vi "Popup window-Cursor value entry.vi"(7 "Waveform Ref in":T3, 10 "Xinformation In":T1, 11 "Timeline Ref in":T5) -> (0 "error out":errorcluster, 1 "Cancelled":bool, 2 "Xinformation Out":T1={"Cursor Span"=0.0, "Icon"=0, "Mouse Down"=FALSE, "Owning VI"=refnum, "Mouse area"=enum."Move", "Dragging"=FALSE, "Drag Offset"=0.0, "Original Cursor Pos"={"Left"=0.0, "Right"=0.0, "Span"=0.0}, "Cursor Redraw"=TRUE}, 3 "Timeline Ref out":T5)   [LabVIEW 2013, in "XGrapher.xctl"]
uses:
  XGrapher.xctl
  Typedefs/Xctrl-Timeline graph ref.ctl
  Typedefs/Xinformation.ctl
  Typedefs/Xcrtl-Click Operation.ctl
  Typedefs/Xctrl-Waveform graph ref.ctl
panel:
  out "Timeline Graph":T4(graph)
  in  "Right Cursor (sec)":dbl min=0.005864328141225338 max=0.085028
  in  "Left Cursor (sec)":dbl min=0.0 max=0.06454358047767395
  in  "Cancel":bool
  in  "OK":bool
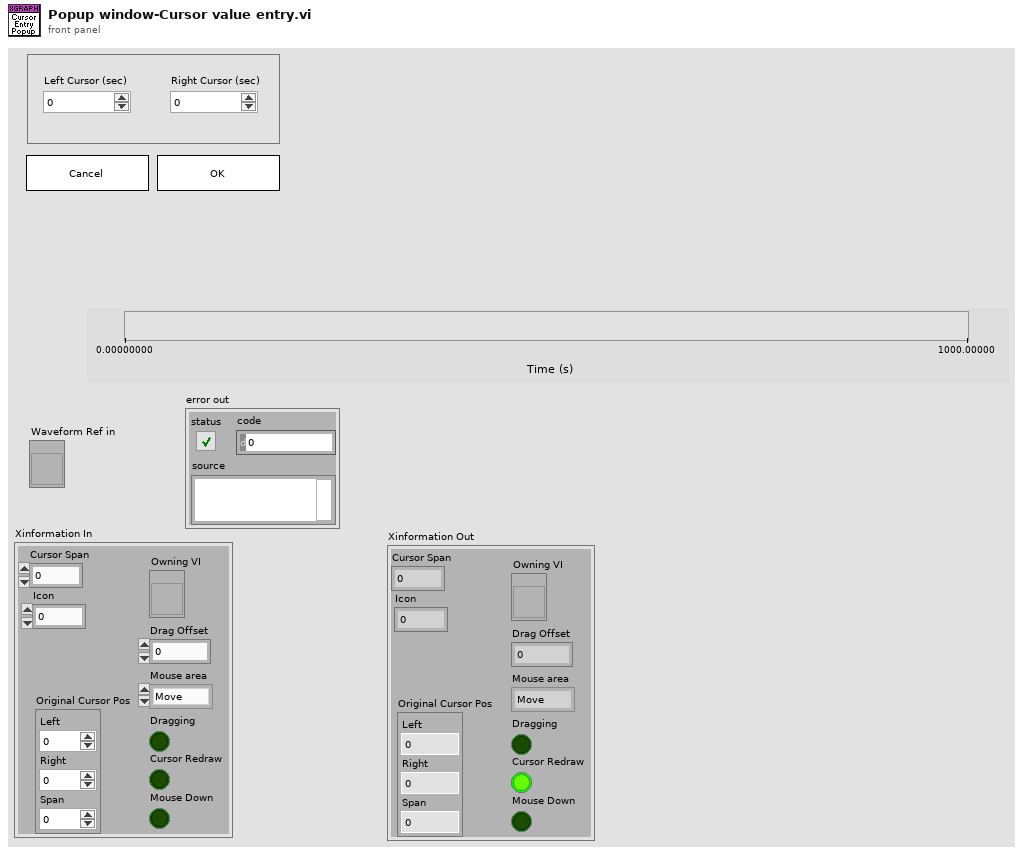
[diagram p1: front panel]
types:
  T1 = typedef "XGrapher.xctl/Xinformation.ctl" = cluster{"Cursor Span":dbl, "Icon":u16, "Mouse Down":bool, "Owning VI":refnum<vi>, "Mouse area":T2, "Dragging":bool, "Drag Offset":dbl, "Original Cursor Pos":cluster{"Left":dbl, "Right":dbl, "Span":dbl}, "Cursor Redraw":bool}
  T2 = typedef "XGrapher.xctl/Xcrtl-Click Operation.ctl" = enum16{"Move", "left cursor", "right cursor", "none"}
  T3 = typedef "XGrapher.xctl/Xctrl-Waveform graph ref.ctl" = refnum<vi>
  T4 = cluster{"X-Axis values":dbl[], "Y-Axis values":dbl[]}[]
  T5 = typedef "XGrapher.xctl/Xctrl-Timeline graph ref.ctl" = refnum<vi>
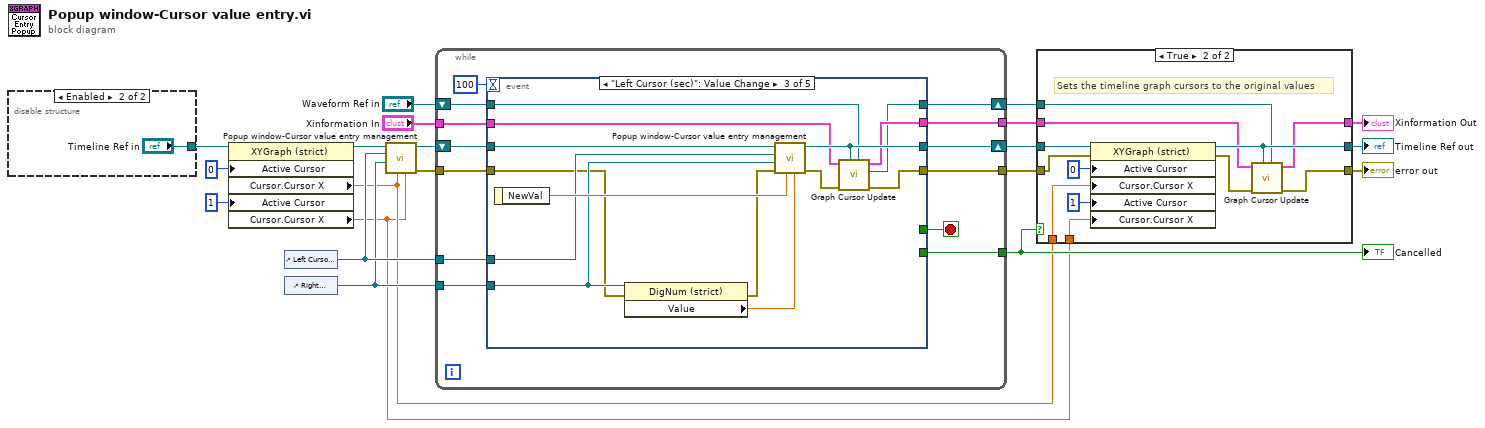
[diagram p0: block diagram]
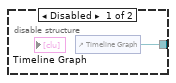
[diagram p3: hidden frame]
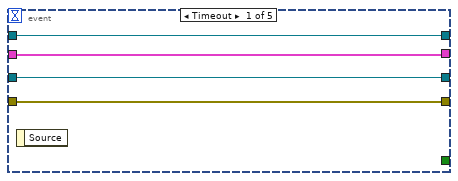
[diagram p4: hidden frame]
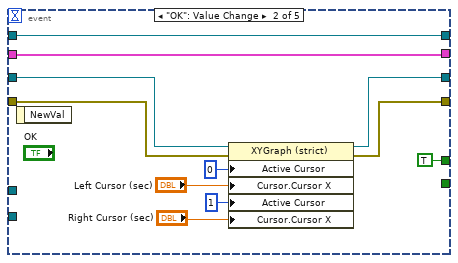
[diagram p5: hidden frame]
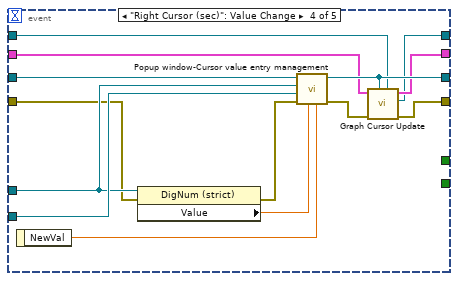
[diagram p6: hidden frame]
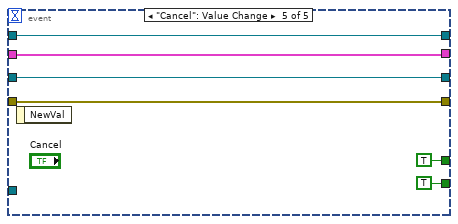
[diagram p7: hidden frame]
diagram:
  n1 = disable-structure shown="Enabled" {
    disable-tunnel: [w21 "Timeline Ref in"] -> w13
    frame Disabled {
      n2 = control-ref of="Timeline Graph"() -> (w21:refnum<vi>)
    }
    frame Enabled {
    }
  }
  n3 = property on="Property Node" class="XYGraph (strict)"(reference=w13, "Active Cursor"=u32 0, "Active Cursor"=u32 1) -> (reference out=w14:T5, "Cursor.Cursor X"=w8:dbl, "Cursor.Cursor X"=w7:dbl)  [unwired: 1 in, 1 out]
  n4 = control-ref of="Left Cursor (sec)"() -> (w18:refnum<vi>)
  n5 = control-ref of="Right Cursor (sec)"() -> (w17:refnum<vi>)
  n6 = call "Popup window-Cursor value entry management.vi"("Rightcursor position"=w7, "Left cursor position"=w8, "Right control ref"=w17, "Left control ref"=w18, "Timeline Ref in"=w14) -> ("error out"=w19:errorcluster, "XYGraph out"=w20:T5)  [unwired: 5 in]
  n7 = while {
    tunnel: [w33] -> w12
    tunnel: w19 -> [w31]
    tunnel: [w30] -> w11
    tunnel: w18 -> [w29]
    tunnel: w17 -> [w28]
    tunnel: "Xinformation In" -> [w26]
    tunnel: [w25] -> w2
    shift-right: [w24] -> w4
    shift-left: w20 -> [w32]
    shift-right: [w23] -> w3
    shift-left: "Waveform Ref in" -> [w27]
    stop <- w34 stop-if-true
    n8 = event shown="[2] \"Left Cursor (sec)\": Value Change" {
      selector: _ -> [_ _ _ _ _]
      dyn-events: _ -> [_ _ _ _ _]
      timeout: 100 -> [_ _ _ _ _]
      tunnel: [_ TRUE ("Cancel") _ _ TRUE ("Cancel")] -> w34
      tunnel: [_ _ _ _ TRUE ("Cancel")] -> w33
      tunnel: w32 -> [w39 w46 w64 w78 w84]
      tunnel: [w39 w45 w57 w69 w84] -> w24
      tunnel: w31 -> [w38 w43 w59 w73 w81]
      tunnel: [w38 w42 w52 w70 w81] -> w30
      tunnel: w29 -> [_ _ w62 w74 _]
      tunnel: w28 -> [_ _ w61 w77 _]
      tunnel: w27 -> [w36 w40 w56 w68 w79]
      tunnel: w26 -> [w37 w41 w55 w67 w80]
      tunnel: [w37 w41 w54 w66 w80] -> w25
      tunnel: [w36 w40 w51 w65 w79] -> w23
      event Timeout {
        n9 = event-data() -> ()  [unwired: 1 in, 1 out]
      }
      event "OK": Value Change {
        n10 = event-data() -> ()  [unwired: 1 in, 1 out]
        n11 = property class="XYGraph (strict)"(reference=w46, error in=w43, "Active Cursor"=u32 0, "Cursor.Cursor X"="Left Cursor (sec)", "Active Cursor"=u32 1, "Cursor.Cursor X"="Right Cursor (sec)") -> (reference out=w45:T5, error out=w42:errorcluster)
      }
      event "Left Cursor (sec)": Value Change {
        n12 = event-data() -> ("NewVal"=w63:dbl)  [unwired: 1 in]
        n13 = property on="Property Node" class="DigNum (strict)"(reference=w61, error in=w59) -> (error out=w58:errorcluster, "Value"=w60:dbl)  [unwired: 1 out]
        n14 = call "Popup window-Cursor value entry management.vi"("Rightcursor position"=w60, "Left cursor position"=w63, "error in"=w58, "Right control ref"=w61, "Left control ref"=w62, "Timeline Ref in"=w64) -> ("error out"=w53:errorcluster, "XYGraph out"=w57:T5)  [unwired: 4 in]
        n15 = call "Graph Cursor Update.vi"("Waveform Ref in"=w56, "Timeline Ref in"=w57, "error in (no error)"=w53, "Xinformation In"=w55) -> ("error out"=w52:errorcluster, "Waveform Ref out"=w51:T3, "Xinformation Out"=w54:T1)  [unwired: 5 in]
      }
      event "Right Cursor (sec)": Value Change {
        n16 = event-data() -> ("NewVal"=w76:dbl)  [unwired: 1 in]
        n17 = property on="Property Node" class="DigNum (strict)"(reference=w74, error in=w73) -> (error out=w72:errorcluster, "Value"=w75:dbl)  [unwired: 1 out]
        n18 = call "Popup window-Cursor value entry management.vi"("Rightcursor position"=w76, "Left cursor position"=w75, "error in"=w72, "Right control ref"=w77, "Left control ref"=w74, "Timeline Ref in"=w78) -> ("error out"=w71:errorcluster, "XYGraph out"=w69:T5)  [unwired: 4 in]
        n19 = call "Graph Cursor Update.vi"("Waveform Ref in"=w68, "Timeline Ref in"=w69, "error in (no error)"=w71, "Xinformation In"=w67) -> ("error out"=w70:errorcluster, "Waveform Ref out"=w65:T3, "Xinformation Out"=w66:T1)  [unwired: 5 in]
      }
      event "Cancel": Value Change {
        n20 = event-data() -> ()  [unwired: 1 in, 1 out]
      }
    }
  }
  "Cancelled" <- w12
  n21 = case shown="True" w12 {
    tunnel: w4 -> [w86 w97]
    tunnel: w11 -> [w87 w96]
    tunnel: [w86 w91] -> w10
    tunnel: [w87 w92] -> w9
    tunnel: w8 -> [_ w95]
    tunnel: w7 -> [_ w94]
    tunnel: w3 -> [_ w90]
    tunnel: w2 -> [w85 w89]
    tunnel: [w85 w88] -> w1
    frame False {
    }
    frame True {
      # "Sets the timeline graph cursors to the original values"
      n22 = property on="Property Node" class="XYGraph (strict)"(reference=w97, error in=w96, "Active Cursor"=u32 0, "Cursor.Cursor X"=w95, "Active Cursor"=u32 1, "Cursor.Cursor X"=w94) -> (reference out=w91:T5, error out=w93:errorcluster)
      n23 = call "Graph Cursor Update.vi"("Waveform Ref in"=w90, "Timeline Ref in"=w91, "error in (no error)"=w93, "Xinformation In"=w89) -> ("error out"=w92:errorcluster, "Xinformation Out"=w88:T1)  [unwired: 5 in, 1 out]
    }
  }
  "Timeline Ref out" <- w10
  "error out" <- w9
  "Xinformation Out" <- w1
